vi "Register For Events.vi"(8 "error in (no error)":errorcluster, 11 "MenuButton Event Handler in":refnum<class "MenuButton Event Handler.lvclass">) -> (0 "error out":errorcluster, 3 "MenuButton Event Handler out":refnum<class "MenuButton Event Handler.lvclass">)   [LabVIEW 2017, in "MenuButtons.lvlib" / "MenuButton Event Handler.lvclass"]
uses:
  MenuButton Event Handler.lvclass
  MenuButton Event Handler.lvclass/MenuButton Event Handler.ctl
  MenuButton/MenuButton.lvclass/MenuButton.ctl
  MenuButton/MenuButton.lvclass
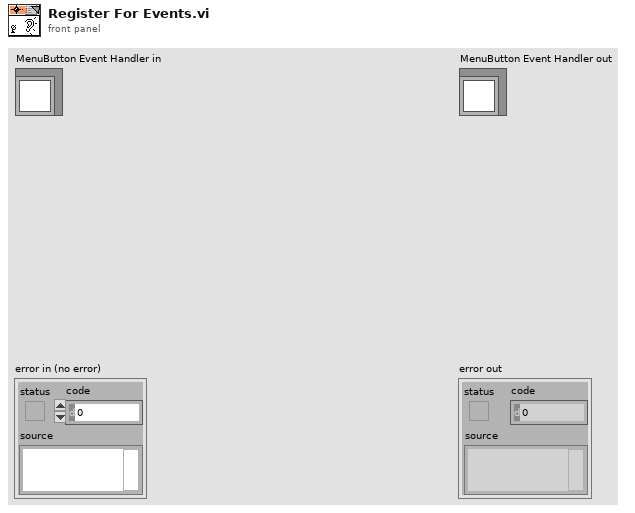
[diagram p1: front panel]
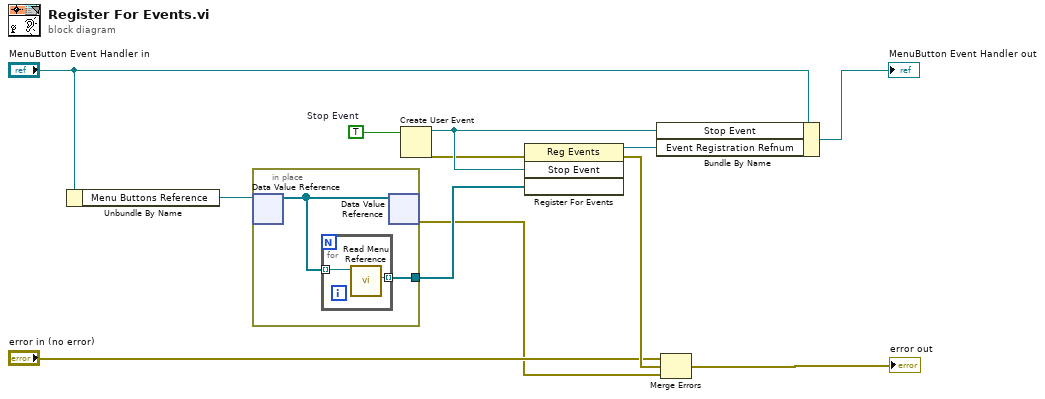
[diagram p0: block diagram]
diagram:
  w12 = TRUE  # Stop Event
  n1 = Unbundle By Name("MenuButton Event Handler in") -> ("Menu Buttons Reference"=w4:refnum<data-value>)
  n2 = in-place {
    in-place-border: [w14] -> w3
    n3 = in-place-dvr #1(w4) -> (w13:refnum<class "MenuButton.lvclass">[])  [unwired: 1 out]
    n4 = for {
      tunnel: [w16] -> w14 mode=indexing
      tunnel: w13 -> [w15] mode=indexing
      n5 = call "Read Menu Reference.vi"("MenuButton in"=w15) -> ("Menu Reference"=w16:refnum<vi>)  [unwired: 8 in, 2 out]
    }
    n6 = in-place-dvr #1(w13) -> (w1:errorcluster)  [unwired: 1 out]
  }
  n7 = Create User Event(user event datatype=w12) -> (user event=w10:refnum<user-event>, error out=w9:errorcluster)  [unwired: 1 in]
  n8 = register-events(error in=w9, w10, w3) -> (reference out=w6:refnum<event-registration>, error out=w7:errorcluster)  [unwired: 1 in]
  n9 = Bundle By Name(cluster="MenuButton Event Handler in", "Stop Event"=w10, "Event Registration Refnum"=w6) -> (→"MenuButton Event Handler out":refnum<class "MenuButton Event Handler.lvclass">)
  n10 = Merge Errors("error in (no error)", w7, w1) -> (→"error out":errorcluster)
